vi "ColorBrewerMaps.vi"(10 "NSeries":i32=1 min=1 max=12 step=1) -> (1 "allPalettes":u32[][](array[colorbox]), 3 "availablePalettes":string[](array[string]))   [LabVIEW 2016]
panel:
  in  "paletteNames":string[](array[string])=["Strong", "Dark", "Light", "Pastel", "Pale", "Brash", "Clean", "Tidy"]
  in  "QualitativeDataSwatches":string[][](array[string])=[["['#7fc97f','#beaed4','#fdc086']", "['#1b9e77','#d95f02','#7570b3']", "['#a6cee3','#1f78b4','#b2df8a']", "['#fbb4ae','#b3cde3','#ccebc5']", "['#b3e2cd','#fdcdac','#cbd5e8']", "['#e41a1c','#377eb8','#4daf4a']", "['#66c2a5','#fc8d62','#8da0cb']", "['#8dd3c7','#ffffb3','#bebada']"], ["['#7fc97f','#beaed4','#fdc086']", "['#1b9e77','#d95f02','#7570b3']", "['#a6cee3','#1f78b4','#b2df8a']", "['#fbb4ae','#b3cde3','#ccebc5']", "['#b3e2cd','#fdcdac','#cbd5e8']", "['#e41a1c','#377eb8','#4daf4a']", "['#66c2a5','#fc8d62','#8da0cb']", "['#8dd3c7','#ffffb3','#bebada']"], ["['#7fc97f','#beaed4','#fdc086']", "['#1b9e77','#d95f02','#7570b3']", "['#a6cee3','#1f78b4','#b2df8a']", "['#fbb4ae','#b3cde3','#ccebc5']", "['#b3e2cd','#fdcdac','#cbd5e8']", "['#e41a1c','#377eb8','#4daf4a']", "['#66c2a5','#fc8d62','#8da0cb']", "['#8dd3c7','#ffffb3','#bebada']"], ["['#7fc97f','#beaed4','#fdc086','#ffff99']", "['#1b9e77','#d95f02','#7570b3','#e7298a']", "['#a6cee3','#1f78b4','#b2df8a','#33a02c']", "['#fbb4ae','#b3cde3','#ccebc5','#decbe4']", "['#b3e2cd','#fdcdac','#cbd5e8','#f4cae4']", "['#e41a1c','#377eb8','#4daf4a','#984ea3']", "['#66c2a5','#fc8d62','#8da0cb','#e78ac3']", "['#8dd3c7','#ffffb3','#bebada','#fb8072']"], ["['#7fc97f','#beaed4','#fdc086','#ffff99','#386cb0']", "['#1b9e77','#d95f02','#7570b3','#e7298a','#66a61e']", "['#a6cee3','#1f78b4','#b2df8a','#33a02c','#fb9a99']", "['#fbb4ae','#b3cde3','#ccebc5','#decbe4','#fed9a6']", "['#b3e2cd','#fdcdac','#cbd5e8','#f4cae4','#e6f5c9']", "['#e41a1c','#377eb8','#4daf4a','#984ea3','#ff7f00']", "['#66c2a5','#fc8d62','#8da0cb','#e78ac3','#a6d854']", "['#8dd3c7','#ffffb3','#bebada','#fb8072','#80b1d3']"], ["['#7fc97f','#beaed4','#fdc086','#ffff99','#386cb0','#f0027f']", "['#1b9e77','#d95f02','#7570b3','#e7298a','#66a61e','#e6ab02']", "['#a6cee3','#1f78b4','#b2df8a','#33a02c','#fb9a99','#e31a1c']", "['#fbb4ae','#b3cde3','#ccebc5','#decbe4','#fed9a6','#ffffcc']", "['#b3e2cd','#fdcdac','#cbd5e8','#f4cae4','#e6f5c9','#fff2ae']", "['#e41a1c','#377eb8','#4daf4a','#984ea3','#ff7f00','#ffff33']", "['#66c2a5','#fc8d62','#8da0cb','#e78ac3','#a6d854','#ffd92f']", "['#8dd3c7','#ffffb3','#bebada','#fb8072','#80b1d3','#fdb462']"], ["['#7fc97f','#beaed4','#fdc086','#ffff99','#386cb0','#f0027f','#bf5b17']", "['#1b9e77','#d95f02','#7570b3','#e7298a','#66a61e','#e6ab02','#a6761d']", "['#a6cee3','#1f78b4','#b2df8a','#33a02c','#fb9a99','#e31a1c','#fdbf6f']", "['#fbb4ae','#b3cde3','#ccebc5','#decbe4','#fed9a6','#ffffcc','#e5d8bd']", "['#b3e2cd','#fdcdac','#cbd5e8','#f4cae4','#e6f5c9','#fff2ae','#f1e2cc']", "['#e41a1c','#377eb8','#4daf4a','#984ea3','#ff7f00','#ffff33','#a65628']", "['#66c2a5','#fc8d62','#8da0cb','#e78ac3','#a6d854','#ffd92f','#e5c494']", "['#8dd3c7','#ffffb3','#bebada','#fb8072','#80b1d3','#fdb462','#b3de69']"], ["['#7fc97f','#beaed4','#fdc086','#ffff99','#386cb0','#f0027f','#bf5b17','#666666']", "['#1b9e77','#d95f02','#7570b3','#e7298a','#66a61e','#e6ab02','#a6761d','#666666']", "['#a6cee3','#1f78b4','#b2df8a','#33a02c','#fb9a99','#e31a1c','#fdbf6f','#ff7f00']", "['#fbb4ae','#b3cde3','#ccebc5','#decbe4','#fed9a6','#ffffcc','#e5d8bd','#fddaec']", "['#b3e2cd','#fdcdac','#cbd5e8','#f4cae4','#e6f5c9','#fff2ae','#f1e2cc','#cccccc']", "['#e41a1c','#377eb8','#4daf4a','#984ea3','#ff7f00','#ffff33','#a65628','#f781bf']", "['#66c2a5','#fc8d62','#8da0cb','#e78ac3','#a6d854','#ffd92f','#e5c494','#b3b3b3']", "['#8dd3c7','#ffffb3','#bebada','#fb8072','#80b1d3','#fdb462','#b3de69','#fccde5']"], ["", "", "['#a6cee3','#1f78b4','#b2df8a','#33a02c','#fb9a99','#e31a1c','#fdbf6f','#ff7f00','#cab2d6']", "['#fbb4ae','#b3cde3','#ccebc5','#decbe4','#fed9a6','#ffffcc','#e5d8bd','#fddaec','#f2f2f2']", "", "['#e41a1c','#377eb8','#4daf4a','#984ea3','#ff7f00','#ffff33','#a65628','#f781bf','#999999']", "", "['#8dd3c7','#ffffb3','#bebada','#fb8072','#80b1d3','#fdb462','#b3de69','#fccde5','#d9d9d9']"], ["", "", "['#a6cee3','#1f78b4','#b2df8a','#33a02c','#fb9a99','#e31a1c','#fdbf6f','#ff7f00','#cab2d6','#6a3d9a']", "", "", "", "", "['#8dd3c7','#ffffb3','#bebada','#fb8072','#80b1d3','#fdb462','#b3de69','#fccde5','#d9d9d9','#bc80bd']"], ["", "", "['#a6cee3','#1f78b4','#b2df8a','#33a02c','#fb9a99','#e31a1c','#fdbf6f','#ff7f00','#cab2d6','#6a3d9a','#ffff99']", "", "", "", "", "['#8dd3c7','#ffffb3','#bebada','#fb8072','#80b1d3','#fdb462','#b3de69','#fccde5','#d9d9d9','#bc80bd','#ccebc5']"], ["", "", "['#a6cee3','#1f78b4','#b2df8a','#33a02c','#fb9a99','#e31a1c','#fdbf6f','#ff7f00','#cab2d6','#6a3d9a','#ffff99','#b15928']", "", "", "", "", "['#8dd3c7','#ffffb3','#bebada','#fb8072','#80b1d3','#fdb462','#b3de69','#fccde5','#d9d9d9','#bc80bd','#ccebc5','#ffed6f']"]]
  # "#ToDo Extend to ColorBrewer Sequential and Diverging schemes"
  # "http://colorbrewer2.org/#type=qualitative&scheme=Accent&n=3"
  # "The contents of the Data Swatches array is copied directly from the ColorBrewer webpage's JS array export option- hence the need to parse"
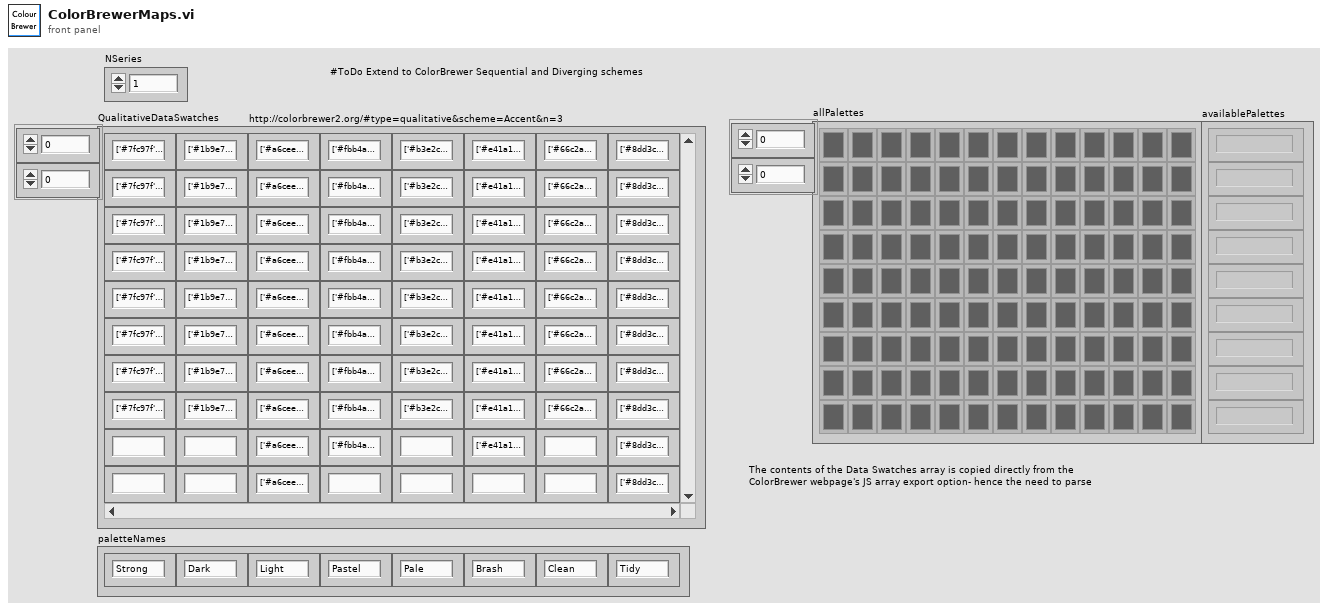
[diagram p1: front panel]
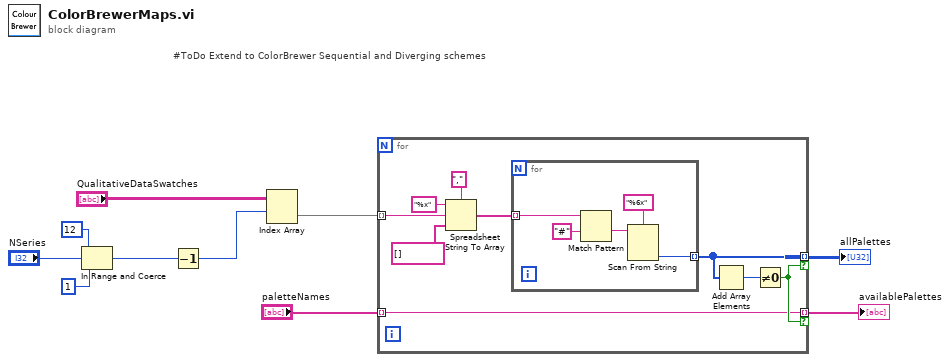
[diagram p0: block diagram]
diagram:
  # "#ToDo Extend to ColorBrewer Sequential and Diverging schemes"
  n1 = In Range and Coerce(upper limit=12, x="NSeries", lower limit=1) -> (coerced(x)=w5:i32)  [unwired: 1 out]
  n2 = Decrement(x=w5) -> (x-1=w8:i32)
  n3 = Index Array(array="QualitativeDataSwatches", index (row)=w8) -> (element=w6:string[])  [unwired: 1 in]
  n4 = for {
    tunnel: [w14] -> w7 mode=indexing if=w12
    tunnel: w6 -> [w15] mode=indexing
    tunnel: [w11] -> w1 mode=indexing if=w12
    tunnel: "paletteNames" -> [w11] mode=indexing
    n5 = Spreadsheet String To Array(delimiter (Tab)=",", format string="%x", spreadsheet string=w15, array type (2D Dbl)=string[] []) -> (array=w16:string[])
    n6 = for {
      tunnel: [w21] -> w14 mode=indexing
      tunnel: w16 -> [w20] mode=indexing
      n7 = Match Pattern(string=w20, regular expression="#") -> (after substring=w23:string)  [unwired: 1 in, 3 out]
      n8 = Scan From String(format string="%6x", input string=w23) -> (output 1=w21:u32)  [unwired: 3 in, 3 out]
    }
    n9 = Add Array Elements(numeric array=w14) -> (sum=w13:u32)
    n10 = Not Equal To 0?(x=w13) -> (x != 0?=w12:bool)
  }
  "allPalettes" <- w7
  "availablePalettes" <- w1
